vi "getDirShellScript.vi"() -> (3 "dirShellScript":path)   [LabVIEW 2018]
doc: "Get the directory of shell script."
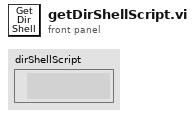
[diagram p1: front panel]
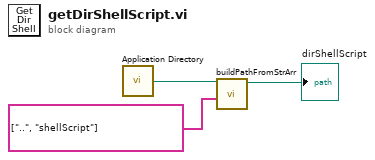
[diagram p0: block diagram]
diagram:
  n1 = call <vilib>:"Application Directory.vi"() -> ("Application Directory"=w3:path)
  n2 = call "buildPathFromStrArr.vi"("String Array"=string[] ["..", "shellScript"], "Root Path"=w3) -> ("Absolute Path"=→"dirShellScript":path)  [unwired: 9 in]
